vi "Close.vi"(8 "error in":errorcluster, 11 "Network Management in":refnum<class "Network Management.lvclass">) -> (0 "error out":errorcluster, 3 "Network Management out":refnum<class "Network Management.lvclass">)   [LabVIEW 2020, in "CANopen.lvlib" / "Network Management.lvlib" / "Network Management.lvclass"]
uses:
  Network Management.lvclass
  Network Management.lvclass/Network Management.ctl
  <vilib>/ActorFramework/Stop Msg/Stop Msg.lvclass
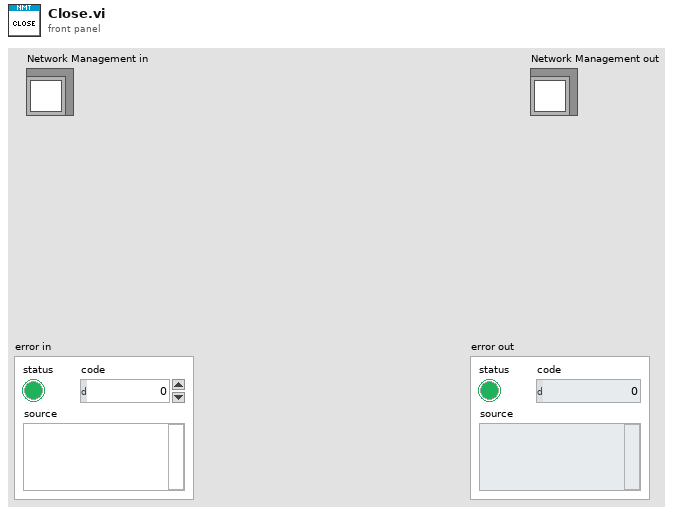
[diagram p1: front panel]
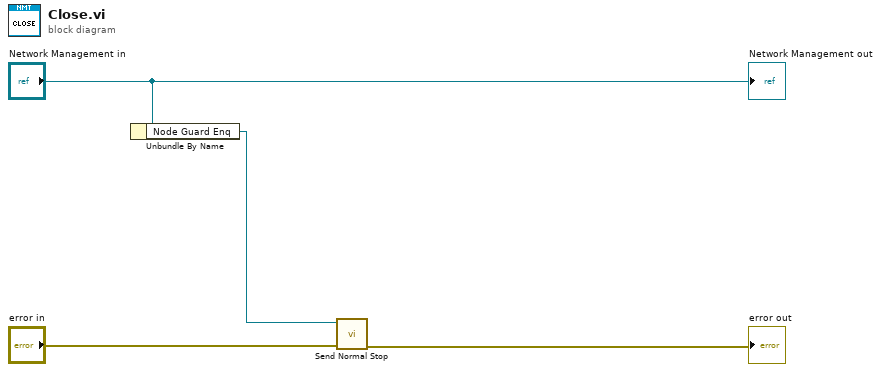
[diagram p0: block diagram]
diagram:
  n1 = Unbundle By Name("Network Management in") -> ("Node Guard Enq"=w2:refnum<class "Message Enqueuer.lvclass">)
  n2 = call <vilib>:"Send Normal Stop.vi"("error in (no error)"="error in", "Message Enqueuer"=w2) -> ("error out"=→"error out":errorcluster)  [unwired: 9 in]
  "Network Management out" <- "Network Management in"
